vi "Spectrometer server.vi"() -> ()   [LabVIEW 2010]
uses:
  <instrlib>/Hamamatsu Spectrometer/Controls/specu1a 1.0.0 Single spectrometer.ctl
  <instrlib>/Hamamatsu Spectrometer/Controls/specu1a 1.0.0 Product Information.ctl
  <instrlib>/Hamamatsu Spectrometer/Controls/specu1a 1.0.0 Single measurement.ctl
  <instrlib>/Hamamatsu Spectrometer/Controls/specu1a 1.0.0 Parameters.ctl
  <instrlib>/Hamamatsu Spectrometer/Controls/specu1a 1.0.0 Trigger Edge.ctl
  <instrlib>/Hamamatsu Spectrometer/Controls/specu1a 1.0.0 Trigger Mode.ctl
  <instrlib>/Hamamatsu Spectrometer/Controls/specu1a 1.0.0 Operation.ctl
  <instrlib>/Hamamatsu Spectrometer/Controls/specu1a 1.0.0 Device interface.ctl
  <instrlib>/Hamamatsu Spectrometer/Controls/specu1a 1.0.0 Model Class.ctl
  <instrlib>/Hamamatsu Spectrometer/Controls/specu1a 1.0.0 Write EEPROM cluster.ctl
panel:
  in  "Dark":bool
  out "Temp time":u32
  in  "Temp":bool
  in  "N mal":u32=10
  out "Measurement time":u32
  in  "Nr of Avgs":i32
  in  "Data":bool
  out "All Spectrometers 2":T1[](array[typedef]) {"White"."Spectrum" format="%.2f"; "Data"."Spectrum" format="%.2f"; "Dark"."Spectrum" format="%.2f"}
  in  "Write Parameters":bool
  in  "Read Parameters":bool
  in  "Cluster":cluster{"Name":string, "Parameters":T4}={"Name"="", "Parameters"={"Integration time"=10000, "Gain"=enum."Low", "TriggerEdge"=enum."Rising", "Trigger Mode"=enum."Internal", "Reserved"=0}}
  in  "stop 2":bool
  in  "Open RC":bool
  in  "Spec. Interface":T7=enum."Open"
  in  "Operations":T8
  in  "All Spectrometers":T1[](array[typedef]) {"White"."Spectrum" format="%.2f"; "Data"."Spectrum" format="%.2f"; "Dark"."Spectrum" format="%.2f"}
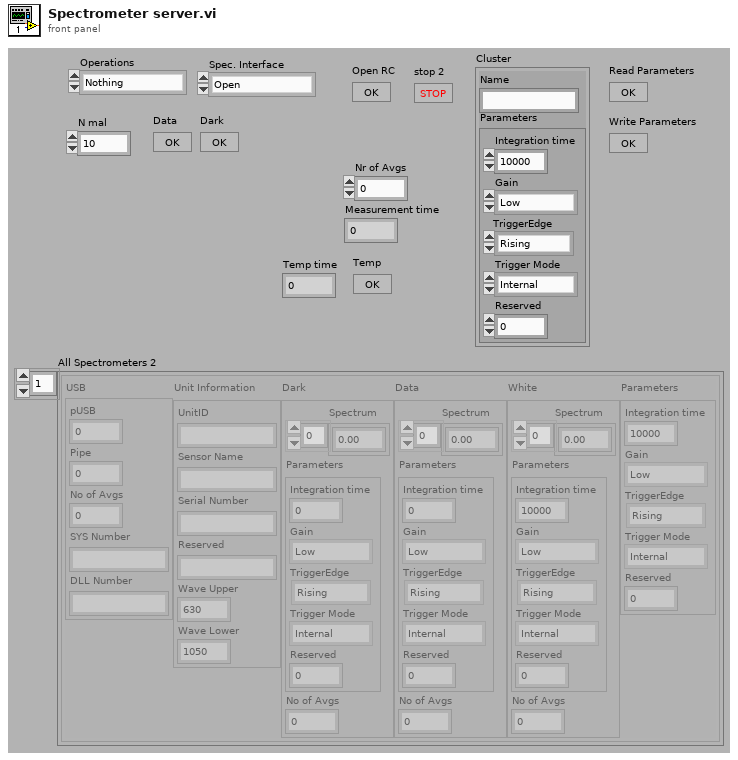
[diagram p1: front panel]
types:
  T1 = typedef "specu1a 1.0.0 Single spectrometer.ctl" = cluster{"USB":cluster{"pUSB":i32, "Pipe":i32, "No of Avgs":u32, "SYS Number":string, "DLL Number":string}, "Unit Information":T2, "Dark":T3, "Data":T3, "White":T3, "Parameters":T4}
  T2 = typedef "specu1a 1.0.0 Product Information.ctl" = cluster{"UnitID":string, "Sensor Name":string, "Serial Number":string, "Reserved":string, "Wave Upper":u16, "Wave Lower":u16}
  T3 = typedef "specu1a 1.0.0 Single measurement.ctl" = cluster{"Spectrum":dbl[], "Parameters":T4, "No of Avgs":u32}
  T4 = typedef "specu1a 1.0.0 Parameters.ctl" = cluster{"Integration time":u32, "Gain":enum16{"Low", "High", "No Function"}, "TriggerEdge":T5, "Trigger Mode":T6, "Reserved":u8}
  T5 = typedef "specu1a 1.0.0 Trigger Edge.ctl" = enum16{"Rising", "Falling", "No Function"}
  T6 = typedef "specu1a 1.0.0 Trigger Mode.ctl" = enum16{"Internal", "Asynchronous", "Synchronous"}
  T7 = typedef "specu1a 1.0.0 Device interface.ctl" = enum16{"Nothing", "Open", "Close", "List", "Status", "Version", "EEPROM", "Product Info", "Parameters", "Temp", "Dark", "White", "Raw", "Spectrum", "Transmission", "Quit"}
  T8 = typedef "specu1a 1.0.0 Operation.ctl" = enum16{"Nothing", "Get DLL Version", "Get SYS Version", "Open Device", "Open pipe", "Read Parameters", "Read PUnit", "Read EEPROM", "Read Status", "Read Calibration", "Read Temperature", "Read Data", "Read Dark", "Read White", "Write Parameters", "Write PUnit", "Write EEPROM", "Write Calibration", "Write Temperature", "Write Data", "Write Dark", "Write White", "Close pipe", "Close Device", "Quit"}
  T9 = cluster{"Spec. Interface":T7, "Name":string, "Variant":variant}
  T10 = cluster{"Operations":T8, "Name":string, "Variant":variant}
  T11 = typedef "specu1a 1.0.0 Model Class.ctl" = enum16{"Invalid", "TG-NIR or SWNIR or UV", "TG-COOLED NIR-I or II", "TM-UV/VIS or VIS/NIR", "TM-UV/VIS or VIS/NIR CCD1 or CCD2", "RC- Vis or SWNIR Module"}
  T12 = typedef "specu1a 1.0.0 Write EEPROM cluster.ctl" = cluster{"Address":u16, "Length":u16, "EEPROM String in":string}
  T13 = typedef "specu1a 1.0.0 Model Name.ctl" = enum16{"Invalid", "TG-NIR", "TG-SWNIR", "TG-UV", "TG-COOLED NIR-II", "TG-COOLED NIR-I", "TM-UV/VIS or VIS/NIR", "TM-UV/VIS or VIS/NIR CCD1", "TM-UV/VIS or VIS/NIR CCD2", "RC-SWNIR Module", "RC-VIS Module"}
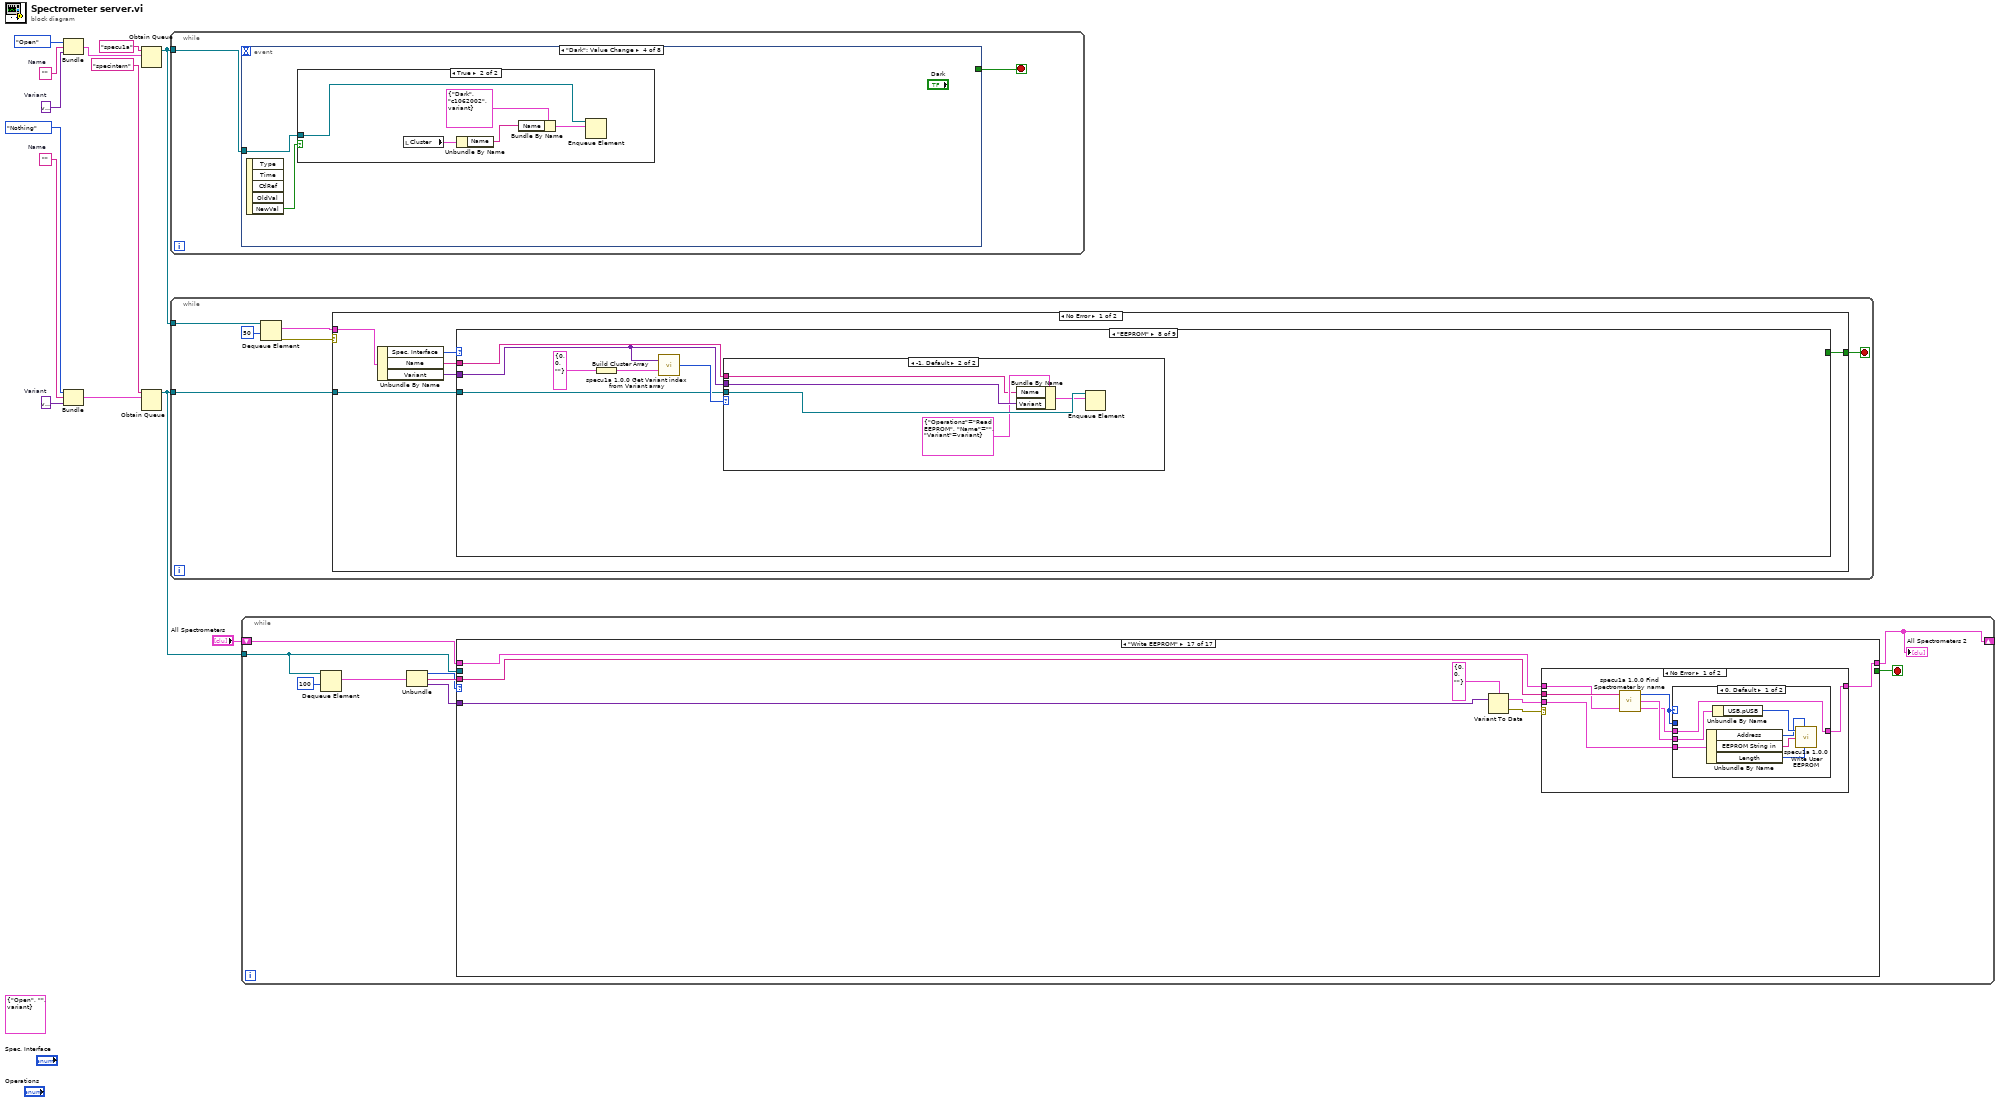
[diagram p0: block diagram]
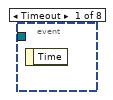
[diagram p2: hidden frame]
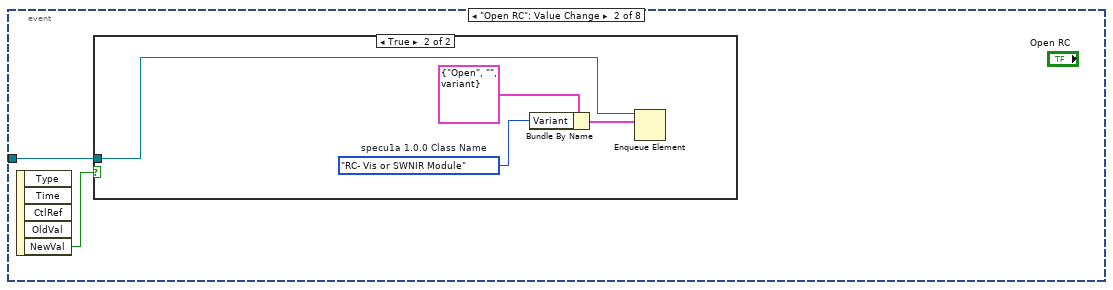
[diagram p3: hidden frame]
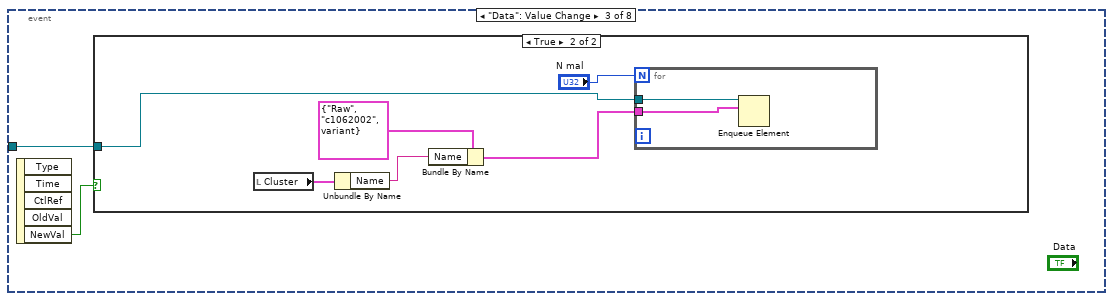
[diagram p5: hidden frame]
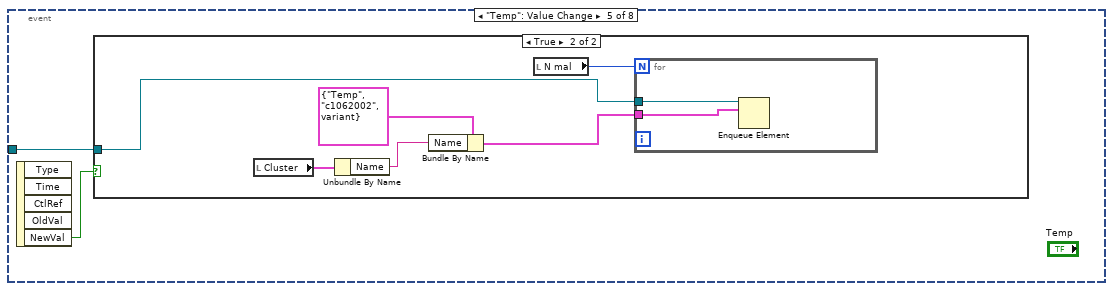
[diagram p8: hidden frame]
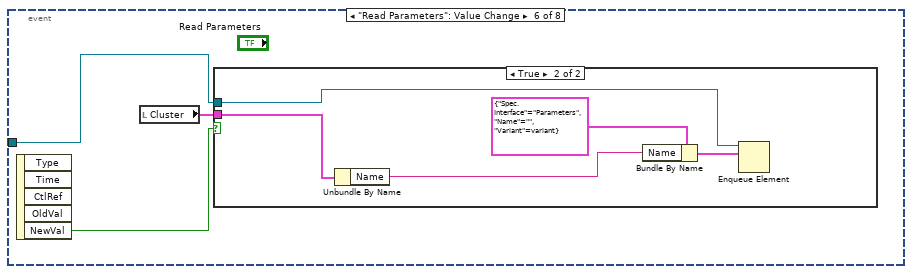
[diagram p10: hidden frame]
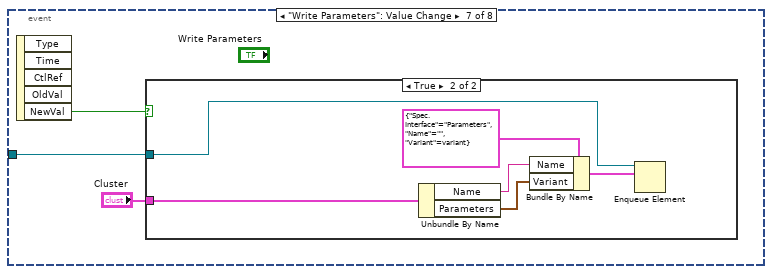
[diagram p12: hidden frame]
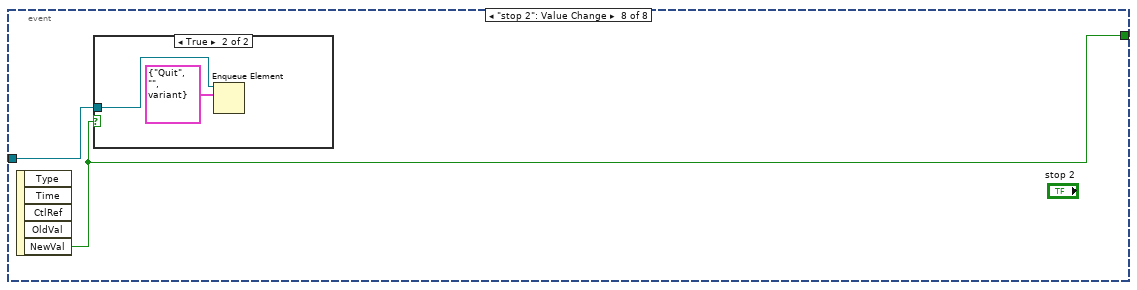
[diagram p14: hidden frame]
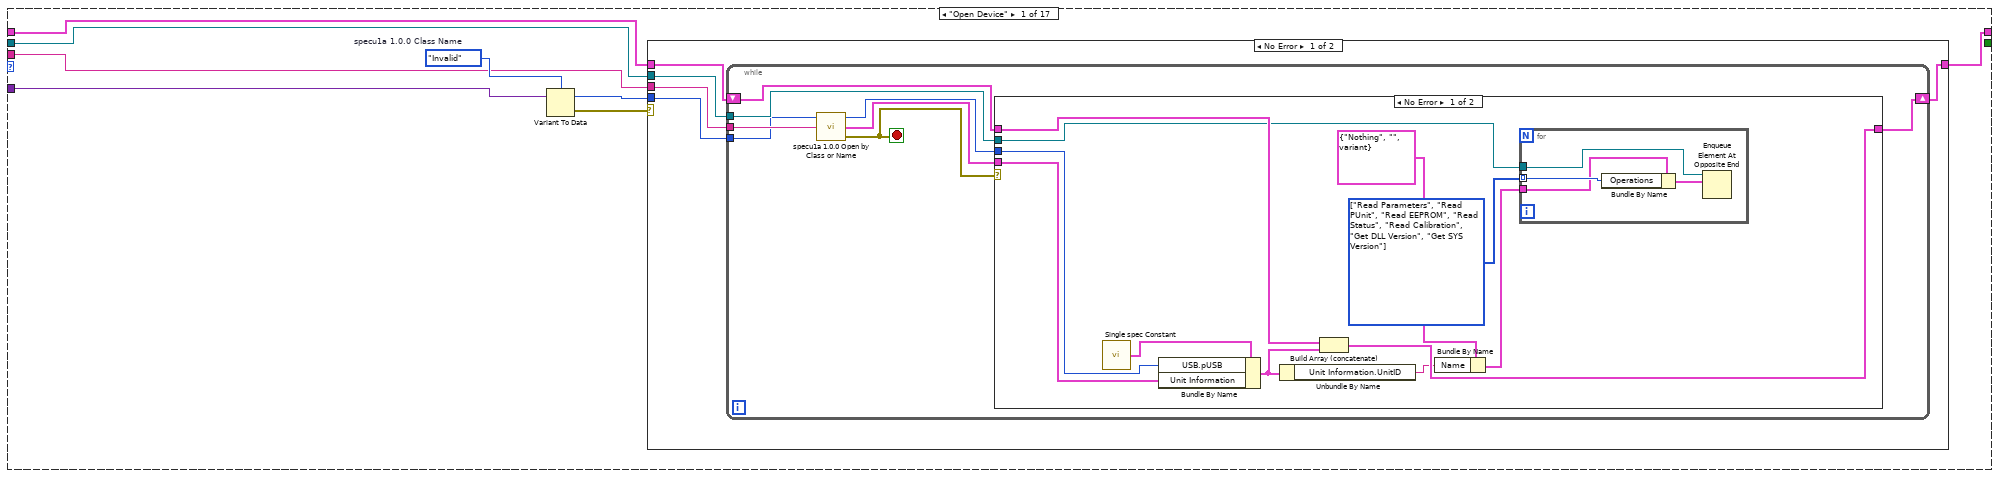
[diagram p16: hidden frame]
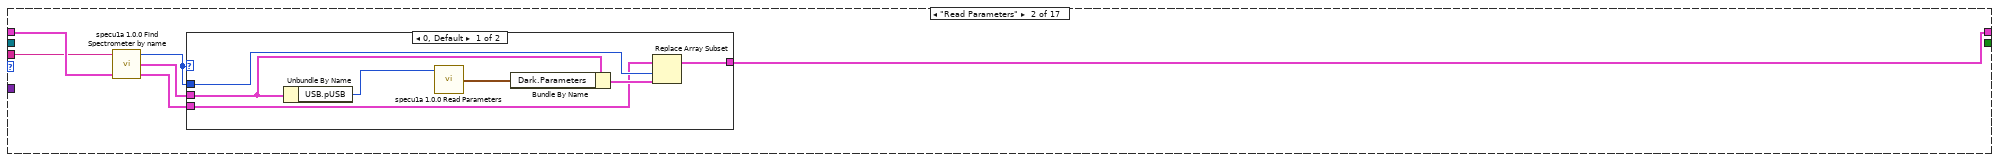
[diagram p19: hidden frame]
diagram:
  w1 = ""  # Name
  (unwired) T9 {"Spec. Interface"=enum."Open", "Name"="", "Variant"=variant} ("output cluster")
  w3 = ""  # Name
  w2 = variant  # Variant
  w4 = variant  # Variant
  n1 = Bundle("Spec. Interface"=specu1a_1.0.0_Device_interface."Open", "Name"=w3, "Variant"=w4) -> (w12:T9)  [unwired: 1 in]
  n2 = Bundle("Operations"=specu1a_1.0.0_Operation."Nothing", "Name"=w1, "Variant"=w2) -> (w7:T10)  [unwired: 1 in]
  n3 = Obtain Queue(name (unnamed)="specu1a", element data type=w12) -> (queue out=w11:refnum<queue>)  [unwired: 3 in, 2 out]
  n4 = Obtain Queue(name (unnamed)="specintern", element data type=w7) -> (queue out=w5:refnum<queue>)  [unwired: 3 in, 2 out]
  n5 = while {
    tunnel: w11 -> [w15]
    stop <- w14 stop-if-true
    n6 = event shown="[3] \"Dark\": Value Change" {
      selector: _ -> [_ _ _ _ _ _ _ _]
      dyn-events: _ -> [_ _ _ _ _ _ _ _]
      timeout: _ -> [_ _ _ _ _ _ _ _]
      tunnel: w15 -> [_ w17 w23 w33 w40 w51 w59 w67]
      tunnel: [_ _ _ _ _ _ _ w66] -> w14
      event Timeout {
        n7 = event-data() -> ()  [unwired: 1 in, 1 out]
      }
      event "Open RC": Value Change {
        n8 = event-data() -> ("NewVal"=w16:bool)  [unwired: 1 in, 4 out]
        n9 = case shown="True" w16 {
          tunnel: w17 -> [_ w20]
          frame False {
          }
          frame True {
            w18 = specu1a_1.0.0_Model_Class."RC- Vis or SWNIR Module"  # specu1a 1.0.0 Class Name
            n10 = Bundle By Name(cluster=T9 {"Spec. Interface"=enum."Open", "Name"="", "Variant"=variant} ("output cluster"), "Variant"=w18) -> (w21:T9)
            n11 = Enqueue Element(queue=w20, element=w21) -> ()  [unwired: 2 in, 3 out]
          }
        }
      }
      event "Data": Value Change {
        n12 = event-data() -> ("NewVal"=w22:bool)  [unwired: 1 in, 4 out]
        n13 = case shown="True" w22 {
          tunnel: w23 -> [_ w28]
          frame False {
          }
          frame True {
            n14 = local read "Cluster"() -> (w26:cluster{"Name":string, "Parameters":T4})
            n15 = Unbundle By Name(w26) -> ("Name"=w25:string)
            n16 = Bundle By Name(cluster=T9 {"Spec. Interface"=enum."Raw", "Name"="c1062002", "Variant"=variant} ("output cluster"), "Name"=w25) -> (w29:T9)
            n17 = for {
              N: "N mal" -> [_]
              tunnel: w29 -> [w31]
              tunnel: w28 -> [w30]
              n18 = Enqueue Element(queue=w30, element=w31) -> ()  [unwired: 2 in, 3 out]
            }
          }
        }
      }
      event "Dark": Value Change {
        n19 = event-data() -> ("NewVal"=w32:bool)  [unwired: 1 in, 4 out]
        n20 = case shown="True" w32 {
          tunnel: w33 -> [_ w37]
          frame False {
          }
          frame True {
            n21 = local read "Cluster"() -> (w35:cluster{"Name":string, "Parameters":T4})
            n22 = Unbundle By Name(w35) -> ("Name"=w34:string)
            n23 = Bundle By Name(cluster=T9 {"Spec. Interface"=enum."Dark", "Name"="c1062002", "Variant"=variant} ("output cluster"), "Name"=w34) -> (w38:T9)
            n24 = Enqueue Element(queue=w37, element=w38) -> ()  [unwired: 2 in, 3 out]
          }
        }
      }
      event "Temp": Value Change {
        n25 = event-data() -> ("NewVal"=w39:bool)  [unwired: 1 in, 4 out]
        n26 = case shown="True" w39 {
          tunnel: w40 -> [_ w45]
          frame False {
          }
          frame True {
            n27 = local read "Cluster"() -> (w43:cluster{"Name":string, "Parameters":T4})
            n28 = Unbundle By Name(w43) -> ("Name"=w42:string)
            n29 = Bundle By Name(cluster=T9 {"Spec. Interface"=enum."Temp", "Name"="c1062002", "Variant"=variant} ("output cluster"), "Name"=w42) -> (w46:T9)
            n30 = local read "N mal"() -> (w41:u32)
            n31 = for {
              N: w41 -> [_]
              tunnel: w46 -> [w48]
              tunnel: w45 -> [w47]
              n32 = Enqueue Element(queue=w47, element=w48) -> ()  [unwired: 2 in, 3 out]
            }
          }
        }
      }
      event "Read Parameters": Value Change {
        n33 = event-data() -> ("NewVal"=w50:bool)  [unwired: 1 in, 4 out]
        n34 = local read "Cluster"() -> (w49:cluster{"Name":string, "Parameters":T4})
        n35 = case shown="True" w50 {
          tunnel: w51 -> [_ w56]
          tunnel: w49 -> [_ w55]
          frame False {
          }
          frame True {
            n36 = Unbundle By Name(w55) -> ("Name"=w54:string)
            n37 = Bundle By Name(cluster=T9 {"Spec. Interface"=enum."Parameters", "Name"="", "Variant"=variant} ("output cluster"), "Name"=w54) -> (w52:T9)
            n38 = Enqueue Element(queue=w56, element=w52) -> ()  [unwired: 2 in, 3 out]
          }
        }
      }
      event "Write Parameters": Value Change {
        n39 = event-data() -> ("NewVal"=w58:bool)  [unwired: 1 in, 4 out]
        n40 = case shown="True" w58 {
          tunnel: w59 -> [_ w64]
          tunnel: "Cluster" -> [_ w62]
          frame False {
          }
          frame True {
            n41 = Unbundle By Name(w62) -> ("Name"=w61:string, "Parameters"=w60:T4)
            n42 = Bundle By Name(cluster=T9 {"Spec. Interface"=enum."Parameters", "Name"="", "Variant"=variant} ("output cluster"), "Name"=w61, "Variant"=w60) -> (w65:T9)
            n43 = Enqueue Element(queue=w64, element=w65) -> ()  [unwired: 2 in, 3 out]
          }
        }
      }
      event "stop 2": Value Change {
        n44 = event-data() -> ("NewVal"=w66:bool)  [unwired: 1 in, 4 out]
        n45 = case shown="True" w66 {
          tunnel: w67 -> [_ w69]
          frame False {
          }
          frame True {
            n46 = Enqueue Element(queue=w69, element=T9 {"Spec. Interface"=enum."Quit", "Name"="", "Variant"=variant} ("output cluster")) -> ()  [unwired: 2 in, 3 out]
          }
        }
      }
    }
  }
  n47 = while {
    tunnel: w11 -> [w72]
    tunnel: w5 -> [w71]
    stop <- w70 stop-if-true
    n48 = Dequeue Element(queue=w72, timeout in ms (-1)=50) -> (element=w73:T9, error out=w74:errorcluster)  [unwired: 1 in, 2 out]
    n49 = case shown="No Error" w74 {
      tunnel: w73 -> [w81 _]
      tunnel: w71 -> [w79 _]
      tunnel: [w78 _] -> w70
      frame No Error {
        n50 = Unbundle By Name(w81) -> ("Spec. Interface"=w77:T7, "Name"=w76:string, "Variant"=w80:variant)
        n51 = case shown="\"EEPROM\"" w77 {
          tunnel: w80 -> [_ w83 w104 w156 w209 w264 w281 w298 _]
          tunnel: w79 -> [_ w84 w105 w157 w210 w263 w280 w297 w314]
          tunnel: [_ _ _ _ _ _ _ _ TRUE] -> w78
          tunnel: w76 -> [_ w82 w103 w155 w208 w261 w279 w296 _]
          frame "Nothing", Default {
          }
          frame "Open" {
            n52 = case shown="\"\"" w82 {
              selector: w82 -> [_ w100]
              tunnel: w84 -> [w87 w102]
              tunnel: w83 -> [w86 w98]
              frame "" {
                w91 = specu1a_1.0.0_Model_Class."Invalid"  # specu1a 1.0.0 Class Name
                n53 = To Variant(anything=w91) -> (Variant=w90:variant)
                n54 = Build Cluster Array(w90) -> (w89:cluster{"Variant":variant}[])
                n55 = call <instrlib>:"specu1a 1.0.0 Get Variant index from Variant array.vi"("Array"=w89, "Variant"=w86) -> ("Numeric"=w88:i32)
                n56 = case shown="0" w88 {
                  tunnel: w87 -> [_ w97]
                  tunnel: w86 -> [_ w96]
                  tunnel: T10 {"Operations"=enum."Open Device", "Name"="", "Variant"=variant} ("element") -> [_ w94]
                  frame -1, Default {
                  }
                  frame 0 {
                    w95 = specu1a_1.0.0_Model_Class."Invalid"  # specu1a 1.0.0 Class Name
                    n57 = Variant To Data(Variant=w96, type=w95) -> (data=w92:T11)  [unwired: 1 in, 1 out]
                    n58 = Bundle By Name(cluster=w94, "Variant"=w92) -> (w93:T10)
                    n59 = Enqueue Element(queue=w97, element=w93) -> ()  [unwired: 2 in, 3 out]
                  }
                }
              }
              frame "True", Default {
                n60 = Bundle By Name(cluster=T10 {"Operations"=enum."Open Device", "Name"="", "Variant"=variant} ("element"), "Name"=w100, "Variant"=w98) -> (w99:T10)
                n61 = Enqueue Element(queue=w102, element=w99) -> ()  [unwired: 2 in, 3 out]
              }
            }
          }
          frame "Dark" {
            n62 = case shown="\"True\", Default" w103 {
              selector: w103 -> [_ w110]
              tunnel: w105 -> [_ w117]
              tunnel: w104 -> [_ w111]
              frame "" {
              }
              frame "True", Default {
                n63 = To Variant(anything=u16[] []) -> (Variant=w116:variant)
                n64 = Build Cluster Array(w116, i32[] [], sgl[] [], dbl[] [], u32[] []) -> (w112:cluster{"Variant":variant}[])
                n65 = call <instrlib>:"specu1a 1.0.0 Get Variant index from Variant array.vi"("Array"=w112, "Variant"=w111) -> ("Numeric"=w109:i32)
                n66 = case shown="4" w109 {
                  tunnel: w111 -> [w124 w131 w138 w144 w151 _]
                  tunnel: w110 -> [w120 w127 w134 w141 w148 w153]
                  tunnel: [w119 w126 w133 w140 w147 w152] -> w108
                  frame 0 {
                    n67 = Variant To Data(Variant=w124, type=u16[] []) -> (data=w122:u16[])  [unwired: 1 in, 1 out]
                    n68 = To Double Precision Float(number=w122) -> (double precision float=w118:dbl[])
                    n69 = Bundle By Name(cluster=T10 {"Operations"=enum."Write Dark", "Name"="", "Variant"=variant} ("element"), "Name"=w120, "Variant"=w118) -> (w119:T10)
                  }
                  frame 1 {
                    n70 = Variant To Data(Variant=w131, type=i32[] []) -> (data=w129:i32[])  [unwired: 1 in, 1 out]
                    n71 = To Double Precision Float(number=w129) -> (double precision float=w125:dbl[])
                    n72 = Bundle By Name(cluster=T10 {"Operations"=enum."Write Dark", "Name"="", "Variant"=variant} ("element"), "Name"=w127, "Variant"=w125) -> (w126:T10)
                  }
                  frame 2 {
                    n73 = Variant To Data(Variant=w138, type=sgl[] []) -> (data=w136:sgl[])  [unwired: 1 in, 1 out]
                    n74 = To Double Precision Float(number=w136) -> (double precision float=w132:dbl[])
                    n75 = Bundle By Name(cluster=T10 {"Operations"=enum."Write Dark", "Name"="", "Variant"=variant} ("element"), "Name"=w134, "Variant"=w132) -> (w133:T10)
                  }
                  frame 3 {
                    n76 = Variant To Data(Variant=w144, type=dbl[] []) -> (data=w139:dbl[])  [unwired: 1 in, 1 out]
                    n77 = Bundle By Name(cluster=T10 {"Operations"=enum."Write Dark", "Name"="", "Variant"=variant} ("element"), "Name"=w141, "Variant"=w139) -> (w140:T10)
                  }
                  frame 4 {
                    n78 = Variant To Data(Variant=w151, type=u32[] []) -> (data=w146:u32[])  [unwired: 1 in, 1 out]
                    n79 = To Double Precision Float(number=w146) -> (double precision float=w145:dbl[])
                    n80 = Bundle By Name(cluster=T10 {"Operations"=enum."Write Dark", "Name"="", "Variant"=variant} ("element"), "Name"=w148, "Variant"=w145) -> (w147:T10)
                  }
                  frame -1, Default {
                    n81 = Bundle By Name(cluster=T10 {"Operations"=enum."Read Dark", "Name"="", "Variant"=variant} ("element"), "Name"=w153) -> (w152:T10)
                  }
                }
                n82 = Enqueue Element(queue=w117, element=w108) -> ()  [unwired: 2 in, 3 out]
              }
            }
          }
          frame "White" {
            n83 = case shown="\"True\", Default" w155 {
              selector: w155 -> [_ w163]
              tunnel: w157 -> [_ w170]
              tunnel: w156 -> [_ w164]
              frame "" {
              }
              frame "True", Default {
                n84 = To Variant(anything=u16[] []) -> (Variant=w169:variant)
                n85 = Build Cluster Array(w169, i32[] [], sgl[] [], dbl[] [], u32[] []) -> (w165:cluster{"Variant":variant}[])
                n86 = call <instrlib>:"specu1a 1.0.0 Get Variant index from Variant array.vi"("Array"=w165, "Variant"=w164) -> ("Numeric"=w162:i32)
                n87 = case shown="-1, Default" w162 {
                  tunnel: w164 -> [w177 w184 w191 w197 w204 _]
                  tunnel: w163 -> [w174 w181 w188 w195 w202 w206]
                  tunnel: [w173 w180 w187 w194 w201 w205] -> w161
                  tunnel: T10 {"Operations"=enum."Write White", "Name"="", "Variant"=variant} ("element") -> [w171 w178 w185 w192 w198 _]
                  frame 0 {
                    n88 = Variant To Data(Variant=w177, type=u16[] []) -> (data=w175:u16[])  [unwired: 1 in, 1 out]
                    n89 = To Double Precision Float(number=w175) -> (double precision float=w172:dbl[])
                    n90 = Bundle By Name(cluster=w171, "Name"=w174, "Variant"=w172) -> (w173:T10)
                  }
                  frame 1 {
                    n91 = Variant To Data(Variant=w184, type=i32[] []) -> (data=w182:i32[])  [unwired: 1 in, 1 out]
                    n92 = To Double Precision Float(number=w182) -> (double precision float=w179:dbl[])
                    n93 = Bundle By Name(cluster=w178, "Name"=w181, "Variant"=w179) -> (w180:T10)
                  }
                  frame 2 {
                    n94 = Variant To Data(Variant=w191, type=sgl[] []) -> (data=w189:sgl[])  [unwired: 1 in, 1 out]
                    n95 = To Double Precision Float(number=w189) -> (double precision float=w186:dbl[])
                    n96 = Bundle By Name(cluster=w185, "Name"=w188, "Variant"=w186) -> (w187:T10)
                  }
                  frame 3 {
                    n97 = Variant To Data(Variant=w197, type=dbl[] []) -> (data=w193:dbl[])  [unwired: 1 in, 1 out]
                    n98 = Bundle By Name(cluster=w192, "Name"=w195, "Variant"=w193) -> (w194:T10)
                  }
                  frame 4 {
                    n99 = Variant To Data(Variant=w204, type=u32[] []) -> (data=w200:u32[])  [unwired: 1 in, 1 out]
                    n100 = To Double Precision Float(number=w200) -> (double precision float=w199:dbl[])
                    n101 = Bundle By Name(cluster=w198, "Name"=w202, "Variant"=w199) -> (w201:T10)
                  }
                  frame -1, Default {
                    n102 = Bundle By Name(cluster=T10 {"Operations"=enum."Read White", "Name"="", "Variant"=variant} ("element"), "Name"=w206) -> (w205:T10)
                  }
                }
                n103 = Enqueue Element(queue=w170, element=w161) -> ()  [unwired: 2 in, 3 out]
              }
            }
          }
          frame "Raw" {
            n104 = case shown="\"True\", Default" w208 {
              selector: w208 -> [_ w221]
              tunnel: w210 -> [_ w223]
              tunnel: w209 -> [_ w222]
              frame "" {
              }
              frame "True", Default {
                n105 = To Variant(anything=u16[] []) -> (Variant=w217:variant)
                n106 = Build Cluster Array(w217, i32[] [], sgl[] [], dbl[] [], u32[] []) -> (w211:cluster{"Variant":variant}[])
                n107 = call <instrlib>:"specu1a 1.0.0 Get Variant index from Variant array.vi"("Array"=w211, "Variant"=w222) -> ("Numeric"=w220:i32)
                n108 = case shown="-1, Default" w220 {
                  tunnel: w222 -> [w230 w237 w244 w250 w257 _]
                  tunnel: w221 -> [w227 w234 w241 w248 w255 w259]
                  tunnel: [w226 w233 w240 w247 w254 w258] -> w219
                  tunnel: T10 {"Operations"=enum."Write Data", "Name"="", "Variant"=variant} ("element") -> [w224 w231 w238 w245 w251 _]
                  frame 0 {
                    n109 = Variant To Data(Variant=w230, type=u16[] []) -> (data=w228:u16[])  [unwired: 1 in, 1 out]
                    n110 = To Double Precision Float(number=w228) -> (double precision float=w225:dbl[])
                    n111 = Bundle By Name(cluster=w224, "Name"=w227, "Variant"=w225) -> (w226:T10)
                  }
                  frame 1 {
                    n112 = Variant To Data(Variant=w237, type=i32[] []) -> (data=w235:i32[])  [unwired: 1 in, 1 out]
                    n113 = To Double Precision Float(number=w235) -> (double precision float=w232:dbl[])
                    n114 = Bundle By Name(cluster=w231, "Name"=w234, "Variant"=w232) -> (w233:T10)
                  }
                  frame 2 {
                    n115 = Variant To Data(Variant=w244, type=sgl[] []) -> (data=w242:sgl[])  [unwired: 1 in, 1 out]
                    n116 = To Double Precision Float(number=w242) -> (double precision float=w239:dbl[])
                    n117 = Bundle By Name(cluster=w238, "Name"=w241, "Variant"=w239) -> (w240:T10)
                  }
                  frame 3 {
                    n118 = Variant To Data(Variant=w250, type=dbl[] []) -> (data=w246:dbl[])  [unwired: 1 in, 1 out]
                    n119 = Bundle By Name(cluster=w245, "Name"=w248, "Variant"=w246) -> (w247:T10)
                  }
                  frame 4 {
                    n120 = Variant To Data(Variant=w257, type=u32[] []) -> (data=w253:u32[])  [unwired: 1 in, 1 out]
                    n121 = To Double Precision Float(number=w253) -> (double precision float=w252:dbl[])
                    n122 = Bundle By Name(cluster=w251, "Name"=w255, "Variant"=w252) -> (w254:T10)
                  }
                  frame -1, Default {
                    n123 = Bundle By Name(cluster=T10 {"Operations"=enum."Read Data", "Name"="", "Variant"=variant} ("element"), "Name"=w259) -> (w258:T10)
                  }
                }
                n124 = Enqueue Element(queue=w223, element=w219) -> ()  [unwired: 2 in, 3 out]
              }
            }
          }
          frame "Parameters" {
            w262 = T4 {"Integration time"=10000, "Gain"=enum."Low", "TriggerEdge"=enum."Rising", "Trigger Mode"=enum."Internal", "Reserved"=0}  # Parameters
            n125 = To Variant(anything=w262) -> (Variant=w267:variant)
            n126 = Build Cluster Array(w267) -> (w266:cluster{"Variant":variant}[])
            n127 = call <instrlib>:"specu1a 1.0.0 Get Variant index from Variant array.vi"("Array"=w266, "Variant"=w264) -> ("Numeric"=w265:i32)
            n128 = case shown="-1, Default" w265 {
              tunnel: w264 -> [w272 w277]
              tunnel: w263 -> [w271 w276]
              tunnel: w261 -> [w269 w274]
              frame 0 {
                n129 = Bundle By Name(cluster=T10 {"Operations"=enum."Write Parameters", "Name"="", "Variant"=variant} ("element"), "Name"=w269, "Variant"=w272) -> (w268:T10)
                n130 = Enqueue Element(queue=w271, element=w268) -> ()  [unwired: 2 in, 3 out]
              }
              frame -1, Default {
                n131 = Bundle By Name(cluster=T10 {"Operations"=enum."Read Parameters", "Name"="", "Variant"=variant} ("element"), "Name"=w274, "Variant"=w277) -> (w273:T10)
                n132 = Enqueue Element(queue=w276, element=w273) -> ()  [unwired: 2 in, 3 out]
              }
            }
          }
          frame "Temp" {
            w278 = 0.0  # Temperature (°C)
            n133 = To Variant(anything=w278) -> (Variant=w284:variant)
            n134 = Build Cluster Array(w284) -> (w283:cluster{"Variant":variant}[])
            n135 = call <instrlib>:"specu1a 1.0.0 Get Variant index from Variant array.vi"("Array"=w283, "Variant"=w281) -> ("Numeric"=w282:i32)
            n136 = case shown="0" w282 {
              tunnel: w281 -> [w289 w294]
              tunnel: w280 -> [w288 w293]
              tunnel: w279 -> [w286 w291]
              frame 0 {
                n137 = Bundle By Name(cluster=T10 {"Operations"=enum."Write Temperature", "Name"="", "Variant"=variant} ("element"), "Name"=w286, "Variant"=w289) -> (w285:T10)
                n138 = Enqueue Element(queue=w288, element=w285) -> ()  [unwired: 2 in, 3 out]
              }
              frame -1, Default {
                n139 = Bundle By Name(cluster=T10 {"Operations"=enum."Read Temperature", "Name"="", "Variant"=variant} ("element"), "Name"=w291, "Variant"=w294) -> (w290:T10)
                n140 = Enqueue Element(queue=w293, element=w290) -> ()  [unwired: 2 in, 3 out]
              }
            }
          }
          frame "EEPROM" {
            n141 = Build Cluster Array(T12 {"Address"=0, "Length"=0, "EEPROM String in"=""} ("output cluster")) -> (w300:cluster{"output cluster":T12}[])
            n142 = call <instrlib>:"specu1a 1.0.0 Get Variant index from Variant array.vi"("Array"=w300, "Variant"=w298) -> ("Numeric"=w299:i32)
            n143 = case shown="-1, Default" w299 {
              tunnel: w298 -> [w305 w310]
              tunnel: w297 -> [w304 w309]
              tunnel: w296 -> [w302 w307]
              frame 0 {
                n144 = Bundle By Name(cluster=T10 {"Operations"=enum."Write EEPROM", "Name"="", "Variant"=variant} ("element"), "Name"=w302, "Variant"=w305) -> (w301:T10)
                n145 = Enqueue Element(queue=w304, element=w301) -> ()  [unwired: 2 in, 3 out]
              }
              frame -1, Default {
                n146 = Bundle By Name(cluster=T10 {"Operations"=enum."Read EEPROM", "Name"="", "Variant"=variant} ("element"), "Name"=w307, "Variant"=w310) -> (w306:T10)
                n147 = Enqueue Element(queue=w309, element=w306) -> ()  [unwired: 2 in, 3 out]
              }
            }
          }
          frame "Quit" {
            n148 = Enqueue Element(queue=w314, element=T10 {"Operations"=enum."Close Device", "Name"="", "Variant"=variant}) -> (queue out=w312:refnum<queue>)  [unwired: 2 in, 2 out]
            n149 = Enqueue Element(queue=w312, element=T10 {"Operations"=enum."Quit", "Name"="", "Variant"=variant}) -> ()  [unwired: 2 in, 3 out]
          }
        }
      }
      frame Error {
      }
    }
  }
  n150 = while {
    shift-right: [w316] -> _
    shift-left: "All Spectrometers" -> [w321]
    tunnel: w5 -> [w319]
    stop <- w317 stop-if-true
    n151 = Dequeue Element(queue=w319, timeout in ms (-1)=100) -> (element=w324:T10)  [unwired: 1 in, 3 out]
    n152 = Unbundle(w324) -> ("Operations"=w322:T8, "Name"=w323:string, "Variant"=w318:variant)
    n153 = case shown="\"Write EEPROM\"" w322 {
      selector: w322 -> [_ _ _ _ _ _ _ _ _ w465 _ _ _ _ _ _ _]
      tunnel: w323 -> [w326 w364 w380 w390 w400 w410 w424 w436 w450 w470 _ w517 w563 _ w581 w606 w630]
      tunnel: w321 -> [w330 w368 w382 w392 w402 w412 w426 w438 w452 w472 w513 w516 w562 w580 w585 w609 w633]
      tunnel: [w329 w367 w381 w391 w401 w411 w425 w437 w451 w471 w513 w515 w561 w580 w584 w608 w632] -> w316
      tunnel: w319 -> [w328 _ _ _ _ _ _ _ _ _ _ _ _ _ _ _ _]
      tunnel: w318 -> [w332 _ _ _ _ _ _ _ _ _ _ w514 w560 _ w582 w607 w631]
      tunnel: [_ _ _ _ _ _ _ _ _ _ _ _ _ TRUE _ _ _] -> w317
      frame "Open Device" {
        w327 = specu1a_1.0.0_Model_Class."Invalid"  # specu1a 1.0.0 Class Name
        n154 = Variant To Data(Variant=w332, type=w327) -> (error out=w331:errorcluster, data=w325:T11)  [unwired: 1 in]
        n155 = case shown="No Error" w331 {
          tunnel: w330 -> [w334 w362]
          tunnel: [w333 w362] -> w329
          tunnel: w328 -> [w337 _]
          tunnel: w326 -> [w336 _]
          tunnel: w325 -> [w335 _]
          frame No Error {
            n156 = while {
              tunnel: w337 -> [w342]
              tunnel: w336 -> [w341]
              tunnel: w335 -> [w340]
              shift-right: [w338] -> w333
              shift-left: w334 -> [w339]
              stop <- w345 stop-if-true
              n157 = call <instrlib>:"specu1a 1.0.0 Open by Class or Name.vi"("Unit ID"=w341, "specu1a 1.0.0 Model Class"=w340) -> ("error out"=w345:errorcluster, "Unit Information out"=w343:T2, "Device Handle"=w344:i32)  [unwired: 1 in]
              n158 = case shown="No Error" w345 {
                tunnel: w344 -> [w354 _]
                tunnel: w343 -> [w346 _]
                tunnel: w339 -> [w356 w361]
                tunnel: [w355 w361] -> w338
                tunnel: w342 -> [w351 _]
                frame No Error {
                  w353 = T8[] [enum."Read Parameters", enum."Read PUnit", enum."Read EEPROM", enum."Read Status", enum."Read Calibration", enum."Get DLL Version", enum."Get SYS Version"] items=["Nothing", "Get DLL Version", "Get SYS Version", "Open Device", "Open pipe", "Read Parameters", "Read PUnit", "Read EEPROM", "Read Status", "Read Calibration", "Read Temperature", "Read Data", "Read Dark", "Read White", "Write Parameters", "Write PUnit", "Write EEPROM", "Write Calibration", "Write Temperature", "Write Data", "Write Dark", "Write White", "Close pipe", "Close Device", "Quit"]
                  n159 = call <instrlib>:"Single spec Constant.vi"() -> ("Single Spectrometer"=w347:T1)
                  n160 = Bundle By Name(cluster=w347, "USB.pUSB"=w354, "Unit Information"=w346) -> (w348:T1)
                  n161 = Unbundle By Name(w348) -> ("Unit Information.UnitID"=w352:string)
                  n162 = Build Array (concatenate)(w356, w348) -> (w355:T1[])
                  n163 = Bundle By Name(cluster=T10 {"Operations"=enum."Nothing", "Name"="", "Variant"=variant} ("element"), "Name"=w352) -> (w350:T10)
                  n164 = for {
                    tunnel: w353 -> [w360] mode=indexing
                    tunnel: w351 -> [w359]
                    tunnel: w350 -> [w358]
                    n165 = Bundle By Name(cluster=w358, "Operations"=w360) -> (w357:T10)
                    n166 = Enqueue Element At Opposite End(queue=w359, element=w357) -> ()  [unwired: 2 in, 3 out]
                  }
                }
                frame Error {
                }
              }
            }
          }
          frame Error {
          }
        }
      }
      frame "Read Parameters" {
        n167 = call <instrlib>:"specu1a 1.0.0 Find Spectrometer by name.vi"("All Spectrometers"=w368, "Name"=w364) -> ("All Spectrometers out"=w363:T1[], "Single Spectrometer"=w366:T1, "index of element"=w365:i32)  [unwired: 1 in]
        n168 = case shown="0, Default" w365 {
          tunnel: w363 -> [w370 w376]
          tunnel: [w369 w376] -> w367
          tunnel: w365 -> [w371 _]
          tunnel: w366 -> [w374 _]
          frame 0, Default {
            n169 = Unbundle By Name(w374) -> ("USB.pUSB"=w375:i32)
            n170 = call <instrlib>:"specu1a 1.0.0 Read Parameters.vi"("Device Handle"=w375) -> ("Parameters"=w373:T4)  [unwired: 2 in, 2 out]
            n171 = Bundle By Name(cluster=w374, "Dark.Parameters"=w373) -> (w372:T1)
            n172 = Replace Array Subset(array=w370, new element=w372, index=w371) -> (w369:T1[])
          }
          frame -1 {
          }
        }
      }
      frame "Read PUnit" {
        n173 = call <instrlib>:"specu1a 1.0.0 Find Spectrometer by name.vi"("All Spectrometers"=w382, "Name"=w380) -> ("All Spectrometers out"=w377:T1[], "Single Spectrometer"=w379:T1, "index of element"=w378:i32)  [unwired: 1 in]
        n174 = case shown="0, Default" w378 {
          tunnel: w377 -> [w383 w386]
          tunnel: [w383 w386] -> w381
          tunnel: w378 -> [_ _]
          tunnel: w379 -> [w384 _]
          frame 0, Default {
            n175 = Unbundle By Name(w384) -> ("USB.pUSB"=w385:i32)
            n176 = call <instrlib>:"specu1a 1.0.0 Read PUnit Information.vi"("Device Handle"=w385) -> ()  [unwired: 2 in, 3 out]
          }
          frame -1 {
          }
        }
      }
      frame "Read EEPROM" {
        n177 = call <instrlib>:"specu1a 1.0.0 Find Spectrometer by name.vi"("All Spectrometers"=w392, "Name"=w390) -> ("All Spectrometers out"=w387:T1[], "Single Spectrometer"=w389:T1, "index of element"=w388:i32)  [unwired: 1 in]
        n178 = case shown="0, Default" w388 {
          tunnel: w387 -> [w393 w396]
          tunnel: [w393 w396] -> w391
          tunnel: w388 -> [_ _]
          tunnel: w389 -> [w394 _]
          frame 0, Default {
            n179 = Unbundle By Name(w394) -> ("USB.pUSB"=w395:i32)
            n180 = call <instrlib>:"specu1a 1.0.0 Read User EEPROM.vi"("Device Handle"=w395) -> ()  [unwired: 4 in, 3 out]
          }
          frame -1 {
          }
        }
      }
      frame "Read Status" {
        n181 = call <instrlib>:"specu1a 1.0.0 Find Spectrometer by name.vi"("All Spectrometers"=w402, "Name"=w400) -> ("All Spectrometers out"=w397:T1[], "Single Spectrometer"=w399:T1, "index of element"=w398:i32)  [unwired: 1 in]
        n182 = case shown="0, Default" w398 {
          tunnel: w397 -> [w403 w406]
          tunnel: [w403 w406] -> w401
          tunnel: w398 -> [_ _]
          tunnel: w399 -> [w404 _]
          frame 0, Default {
            n183 = Unbundle By Name(w404) -> ("USB.pUSB"=w405:i32)
            n184 = call <instrlib>:"specu1a 1.0.0 Read Status request.vi"("Device Handle"=w405) -> ()  [unwired: 2 in, 3 out]
          }
          frame -1 {
          }
        }
      }
      frame "Read Calibration" {
        n185 = call <instrlib>:"specu1a 1.0.0 Find Spectrometer by name.vi"("All Spectrometers"=w412, "Name"=w410) -> ("All Spectrometers out"=w407:T1[], "Single Spectrometer"=w409:T1, "index of element"=w408:i32)  [unwired: 1 in]
        n186 = case shown="0, Default" w408 {
          tunnel: w407 -> [w413 w416]
          tunnel: [w413 w416] -> w411
          tunnel: w408 -> [_ _]
          tunnel: w409 -> [w414 _]
          frame 0, Default {
            n187 = Unbundle By Name(w414) -> ("USB.pUSB"=w415:i32)
            n188 = call <instrlib>:"specu1a 1.0.0 Read Calibration.vi"("Device Handle"=w415) -> ()  [unwired: 2 in, 3 out]
          }
          frame -1 {
          }
        }
      }
      frame "Read Temperature" {
        n189 = call <instrlib>:"specu1a 1.0.0 Find Spectrometer by name.vi"("All Spectrometers"=w426, "Name"=w424) -> ("All Spectrometers out"=w421:T1[], "Single Spectrometer"=w423:T1, "index of element"=w422:i32)  [unwired: 1 in]
        n190 = for {
          N: 1 -> [_]
          shift-right: [w428] -> w420
          shift-left: _ -> [w427]
          tunnel: [w427] -> w419
          n191 = Tick Count (ms)() -> (millisecond timer value=w428:u32)
        }
        n192 = case shown="0, Default" w422 {
          tunnel: w421 -> [w429 w432]
          tunnel: [w429 w432] -> w425
          tunnel: w422 -> [_ _]
          tunnel: w423 -> [w430 _]
          frame 0, Default {
            n193 = Unbundle By Name(w430) -> ("USB.pUSB"=w431:i32)
            n194 = call <instrlib>:"specu1a 1.0.0 Read Temperature.vi"("Device Handle"=w431) -> ()  [unwired: 2 in, 3 out]
          }
          frame -1 {
          }
        }
        n195 = Subtract(x=w420, y=w419) -> (x-y=→"Temp time":u32)
      }
      frame "Get DLL Version" {
        n196 = call <instrlib>:"specu1a 1.0.0 Find Spectrometer by name.vi"("All Spectrometers"=w438, "Name"=w436) -> ("All Spectrometers out"=w433:T1[], "Single Spectrometer"=w435:T1, "index of element"=w434:i32)  [unwired: 1 in]
        n197 = case shown="0, Default" w434 {
          tunnel: w433 -> [w445 w446]
          tunnel: [w443 w446] -> w437
          tunnel: w434 -> [w440 _]
          tunnel: w435 -> [w442 _]
          frame 0, Default {
            n198 = Unbundle By Name(w442) -> ("USB.pUSB"=w444:i32)
            n199 = call <instrlib>:"specu1a 1.0.0 Read DLL version.vi"("Device Handle"=w444) -> ("DLL Version"=w439:string)  [unwired: 2 in, 2 out]
            n200 = Bundle By Name(cluster=w442, "USB.DLL Number"=w439) -> (w441:T1)
            n201 = Replace Array Subset(array=w445, new element=w441, index=w440) -> (w443:T1[])
          }
          frame -1 {
          }
        }
      }
      frame "Get SYS Version" {
        n202 = call <instrlib>:"specu1a 1.0.0 Find Spectrometer by name.vi"("All Spectrometers"=w452, "Name"=w450) -> ("All Spectrometers out"=w447:T1[], "Single Spectrometer"=w449:T1, "index of element"=w448:i32)  [unwired: 1 in]
        n203 = case shown="0, Default" w448 {
          tunnel: w447 -> [w459 w460]
          tunnel: [w457 w460] -> w451
          tunnel: w448 -> [w454 _]
          tunnel: w449 -> [w456 _]
          frame 0, Default {
            n204 = Unbundle By Name(w456) -> ("USB.pUSB"=w458:i32)
            n205 = call <instrlib>:"specu1a 1.0.0 Read SYS version.vi"("Device Handle"=w458) -> ("SYS Version"=w453:string)  [unwired: 2 in, 2 out]
            n206 = Bundle By Name(cluster=w456, "USB.SYS Number"=w453) -> (w455:T1)
            n207 = Replace Array Subset(array=w459, new element=w455, index=w454) -> (w457:T1[])
          }
          frame -1 {
          }
        }
      }
      frame "Read Data".."Read White" {
        n208 = call <instrlib>:"specu1a 1.0.0 Find Spectrometer by name.vi"("All Spectrometers"=w472, "Name"=w470) -> ("All Spectrometers out"=w467:T1[], "Single Spectrometer"=w469:T1, "index of element"=w468:i32)  [unwired: 1 in]
        n209 = for {
          N: 1 -> [_]
          shift-right: [w474] -> w464
          shift-left: _ -> [w473]
          tunnel: [w473] -> w463
          n210 = Tick Count (ms)() -> (millisecond timer value=w474:u32)
        }
        n211 = case shown="0, Default" w468 {
          tunnel: w467 -> [w488 w512]
          tunnel: [w487 w512] -> w471
          tunnel: w468 -> [w486 _]
          tunnel: w469 -> [w490 _]
          tunnel: T3 {"Spectrum"=[], "Parameters"={"Integration time"=10000, "Gain"=enum."Low", "TriggerEdge"=enum."Rising", "Trigger Mode"=enum."Internal", "Reserved"=0}, "No of Avgs"=0} ("Dark") -> [w491 _]
          tunnel: w465 -> [w484 _]
          frame 0, Default {
            n212 = Unbundle By Name(w490) -> ("Dark.Parameters"=w476:T4, "Unit Information"=w492:T2, "USB.pUSB"=w483:i32)
            n213 = call <instrlib>:"specu1a 1.0.0 Open Pipe.vi"("Device Handle"=w483) -> ("error out"=w477:errorcluster, "Pipe Handle"=w481:i32, "Device Handle out"=w482:i32)  [unwired: 2 in]
            n214 = call <instrlib>:"specu1a 1.0.0 Read Sensor Data.vi"("Device Handle"=w482, "Unit Information"=w492, "Pipe Handle"=w481, "error in (no error)"=w477, "Nr of Averages"="Nr of Avgs") -> ("Device Handle out"=w480:i32, "Pipe Handle out"=w479:i32, "Sensor Data"=w475:dbl[], "error out"=w478:errorcluster)  [unwired: 1 in]
            n215 = call <instrlib>:"specu1a 1.0.0 Close Pipe.vi"("error in (no error)"=w478, "Pipe Handle"=w479, "Device Handle"=w480) -> ()  [unwired: 1 in, 2 out]
            n216 = Bundle By Name(cluster=w491, "Parameters"=w476, "Spectrum"=w475, "No of Avgs"="Nr of Avgs") -> (w489:T3)
            n217 = case shown="\"Read Data\"" w484 {
              tunnel: w490 -> [w498 w504 w510 _]
              tunnel: w489 -> [w497 w503 w509 _]
              tunnel: w488 -> [w495 w501 w507 w511]
              tunnel: [w494 w500 w506 w511] -> w487
              tunnel: w486 -> [w493 w499 w505 _]
              frame "Read White" {
                n218 = Bundle By Name(cluster=w498, "White"=w497) -> (w496:T1)
                n219 = Replace Array Subset(array=w495, new element=w496, index=w493) -> (w494:T1[])
              }
              frame "Read Data" {
                n220 = Bundle By Name(cluster=w504, "Data"=w503) -> (w502:T1)
                n221 = Replace Array Subset(array=w501, new element=w502, index=w499) -> (w500:T1[])
              }
              frame "Read Dark" {
                n222 = Bundle By Name(cluster=w510, "Dark"=w509) -> (w508:T1)
                n223 = Replace Array Subset(array=w507, new element=w508, index=w505) -> (w506:T1[])
              }
              frame "Nothing", Default {
              }
            }
          }
          frame -1 {
          }
        }
        n224 = Subtract(x=w464, y=w463) -> (x-y=→"Measurement time":u32)
      }
      frame "Nothing", Default {
      }
      frame "Close Device" {
        n225 = case shown="\"\"" w517 {
          selector: w517 -> [w523 _]
          tunnel: w516 -> [w522 w537]
          tunnel: [w518 w536] -> w515
          tunnel: w514 -> [_ w535]
          frame "True", Default {
            n226 = call <instrlib>:"specu1a 1.0.0 Find Spectrometer by name.vi"("All Spectrometers"=w522, "Name"=w523) -> ("All Spectrometers out"=w519:T1[], "Single Spectrometer"=w521:T1, "index of element"=w520:i32)  [unwired: 1 in]
            n227 = case shown="0, Default" w520 {
              selector: w520 -> [_ w526]
              tunnel: w521 -> [_ w531]
              tunnel: w519 -> [w524 w527]
              tunnel: [w524 w525] -> w518
              frame -1 {
              }
              frame 0, Default {
                n228 = Unbundle By Name(w531) -> ("USB.pUSB"=w528:i32, "USB.Pipe"=w529:i32)
                n229 = call <instrlib>:"specu1a 1.0.0 Close Pipe.vi"("Device Handle"=w529) -> ("error out"=w530:errorcluster)  [unwired: 3 in, 1 out]
                n230 = call <instrlib>:"specu1a 1.0.0 Close Device.vi"("error in (no error)"=w530, "Device Handle"=w528) -> ()  [unwired: 3 in, 1 out]
                n231 = Delete From Array(array=w527, index=w526) -> (array with subset deleted=w525:T1[])  [unwired: 1 in, 1 out]
              }
            }
          }
          frame "" {
            w534 = specu1a_1.0.0_Model_Class."Invalid"  # specu1a 1.0.0 Class Name
            n232 = Variant To Data(Variant=w535, type=w534) -> (error out=w533:errorcluster, data=w532:T11)  [unwired: 1 in]
            n233 = case shown="Error" w533 {
              tunnel: w537 -> [w541 w546]
              tunnel: [w538 w544] -> w536
              tunnel: w532 -> [_ w545]
              frame Error {
                n234 = for {
                  tunnel: w541 -> [w543] mode=indexing
                  n235 = Unbundle By Name(w543) -> ("USB.pUSB"=w542:i32)
                  n236 = call <instrlib>:"specu1a 1.0.0 Close Device.vi"("Device Handle"=w542) -> ()  [unwired: 4 in, 1 out]
                }
                n237 = call <instrlib>:"Single spec Constant.vi"() -> ("Single Spectrometer"=w540:T1)
                n238 = Initialize Array(w540, 0 ("dimension size")) -> (w538:T1[])
              }
              frame No Error {
                n239 = for {
                  tunnel: w546 -> [w553] mode=indexing
                  tunnel: w545 -> [w550]
                  shift-right: [w547] -> w544
                  shift-left: _ -> [w548]
                  n240 = Unbundle By Name(w553) -> ("Unit Information.UnitID"=w552:string)
                  n241 = call <instrlib>:"specu1a 1.0.0 Unit ID to Device Type.vi"("Unit ID"=w552) -> ("specu1a 1.0.0 Model Name out"=w551:T13)  [unwired: 3 in, 1 out]
                  n242 = Equal?(x=w550, y=w551) -> (x = y?=w549:bool)
                  n243 = case shown="False" w549 {
                    tunnel: w553 -> [w555 w558]
                    tunnel: w548 -> [w556 w557]
                    tunnel: [w554 w557] -> w547
                    frame False {
                      n244 = Build Array (concatenate)(w556, w555) -> (w554:T1[])
                    }
                    frame True {
                      n245 = Unbundle By Name(w558) -> ("USB.pUSB"=w559:i32)
                      n246 = call <instrlib>:"specu1a 1.0.0 Close Device.vi"("Device Handle"=w559) -> ()  [unwired: 4 in, 1 out]
                    }
                  }
                }
              }
            }
          }
        }
      }
      frame "Open pipe" {
        n247 = case shown="\"True\", Default" w563 {
          selector: w563 -> [w569 _]
          tunnel: w562 -> [w564 w578]
          tunnel: [w565 w578] -> w561
          tunnel: w560 -> [_ _]
          frame "True", Default {
            n248 = call <instrlib>:"specu1a 1.0.0 Find Spectrometer by name.vi"("All Spectrometers"=w564, "Name"=w569) -> ("All Spectrometers out"=w566:T1[], "Single Spectrometer"=w568:T1, "index of element"=w567:i32)  [unwired: 1 in]
            n249 = case shown="0, Default" w567 {
              selector: w567 -> [_ w574]
              tunnel: w568 -> [_ w577]
              tunnel: w566 -> [w570 w571]
              tunnel: [w570 w572] -> w565
              frame -1 {
              }
              frame 0, Default {
                n250 = Unbundle By Name(w577) -> ("USB.pUSB"=w576:i32)
                n251 = call <instrlib>:"specu1a 1.0.0 Open Pipe.vi"("Device Handle"=w576) -> ("Pipe Handle"=w575:i32)  [unwired: 2 in, 2 out]
                n252 = Bundle By Name(cluster=w577, "USB.Pipe"=w575) -> (w573:T1)
                n253 = Replace Array Subset(array=w571, new element=w573, index=w574) -> (w572:T1[])
              }
            }
          }
          frame "" {
          }
        }
      }
      frame "Quit" {
      }
      frame "Write Parameters" {
        w583 = T4 {"Integration time"=10000, "Gain"=enum."Low", "TriggerEdge"=enum."Rising", "Trigger Mode"=enum."Internal", "Reserved"=0}  # Parameters
        n254 = Variant To Data(Variant=w582, type=w583) -> (error out=w587:errorcluster, data=w586:T4)  [unwired: 1 in]
        n255 = case shown="No Error" w587 {
          tunnel: w586 -> [w591 _]
          tunnel: w585 -> [w589 w604]
          tunnel: [w594 w604] -> w584
          tunnel: w581 -> [w590 _]
          frame No Error {
            n256 = call <instrlib>:"specu1a 1.0.0 Find Spectrometer by name.vi"("All Spectrometers"=w589, "Name"=w590) -> ("All Spectrometers out"=w588:T1[], "Single Spectrometer"=w593:T1, "index of element"=w592:i32)  [unwired: 1 in]
            n257 = case shown="0, Default" w592 {
              tunnel: w588 -> [w602 w603]
              tunnel: [w600 w603] -> w594
              tunnel: w592 -> [w599 _]
              tunnel: w593 -> [w598 _]
              tunnel: w591 -> [w595 _]
              frame 0, Default {
                n258 = Unbundle By Name(w598) -> ("USB.pUSB"=w601:i32)
                n259 = call <instrlib>:"specu1a 1.0.0 Write Parameters.vi"("Parameters"=w595, "Device Handle"=w601) -> ("Parameters out"=w597:T4)  [unwired: 1 in, 2 out]
                n260 = Bundle By Name(cluster=w598, "Parameters"=w597) -> (w596:T1)
                n261 = Replace Array Subset(array=w602, new element=w596, index=w599) -> (w600:T1[])
              }
              frame -1 {
              }
            }
          }
          frame Error {
          }
        }
      }
      frame "Write PUnit" {
        n262 = Variant To Data(Variant=w607, type=T2 {"UnitID"="", "Sensor Name"="", "Serial Number"="", "Reserved"="", "Wave Upper"=630, "Wave Lower"=1050} ("Unit Information")) -> (error out=w611:errorcluster, data=w610:T2)  [unwired: 1 in]
        n263 = case shown="No Error" w611 {
          tunnel: w610 -> [w615 _]
          tunnel: w609 -> [w613 w628]
          tunnel: [w618 w628] -> w608
          tunnel: w606 -> [w614 _]
          frame No Error {
            n264 = call <instrlib>:"specu1a 1.0.0 Find Spectrometer by name.vi"("All Spectrometers"=w613, "Name"=w614) -> ("All Spectrometers out"=w612:T1[], "Single Spectrometer"=w617:T1, "index of element"=w616:i32)  [unwired: 1 in]
            n265 = case shown="0, Default" w616 {
              tunnel: w612 -> [w626 w627]
              tunnel: [w624 w627] -> w618
              tunnel: w616 -> [w623 _]
              tunnel: w617 -> [w622 _]
              tunnel: w615 -> [w619 _]
              frame 0, Default {
                n266 = Unbundle By Name(w622) -> ("USB.pUSB"=w625:i32)
                n267 = call <instrlib>:"specu1a 1.0.0 Write PUnit Information.vi"("Device Handle"=w625, "P Info in"=w619) -> ("P Info out"=w621:T2)  [unwired: 3 in, 2 out]
                n268 = Bundle By Name(cluster=w622, "Unit Information"=w621) -> (w620:T1)
                n269 = Replace Array Subset(array=w626, new element=w620, index=w623) -> (w624:T1[])
              }
              frame -1 {
              }
            }
          }
          frame Error {
          }
        }
      }
      frame "Write EEPROM" {
        n270 = Variant To Data(Variant=w631, type=T12 {"Address"=0, "Length"=0, "EEPROM String in"=""} ("output cluster")) -> (error out=w635:errorcluster, data=w634:T12)  [unwired: 1 in]
        n271 = case shown="No Error" w635 {
          tunnel: w634 -> [w639 _]
          tunnel: w633 -> [w637 w651]
          tunnel: [w642 w651] -> w632
          tunnel: w630 -> [w638 _]
          frame No Error {
            n272 = call <instrlib>:"specu1a 1.0.0 Find Spectrometer by name.vi"("All Spectrometers"=w637, "Name"=w638) -> ("All Spectrometers out"=w636:T1[], "Single Spectrometer"=w641:T1, "index of element"=w640:i32)  [unwired: 1 in]
            n273 = case shown="0, Default" w640 {
              tunnel: w636 -> [w645 w650]
              tunnel: [w645 w650] -> w642
              tunnel: w640 -> [_ _]
              tunnel: w641 -> [w646 _]
              tunnel: w639 -> [w648 _]
              frame 0, Default {
                n274 = Unbundle By Name(w648) -> ("Address"=w647:u16, "EEPROM String in"=w643:string, "Length"=w644:u16)
                n275 = Unbundle By Name(w646) -> ("USB.pUSB"=w649:i32)
                n276 = call <instrlib>:"specu1a 1.0.0 Write User EEPROM.vi"("Device Handle"=w649, "Address"=w647, "EEPROM String in"=w643, "Length"=w644) -> ()  [unwired: 1 in, 3 out]
              }
              frame -1 {
              }
            }
          }
          frame Error {
          }
        }
      }
    }
    "All Spectrometers 2" <- w316
  }
